vi "load_project.vi"(7 "lv-builder in":refnum<class "lv-builder.lvclass">, 8 "error in (no error)":errorcluster, 11 "project_file":path) -> (0 "error out":errorcluster, 1 "config":T3, 2 "lv-builder out":refnum<class "lv-builder.lvclass">, 3 "build_spec_info []":T1[](array[typedef]), 4 "commit_hash":string)   [LabVIEW 2015, in "lv-build-interface.lvlib"]
uses:
  lv-build-interface.lvlib
  lv-builder/class/lv-builder.lvclass
  lv-build/public/_controls/configuration.ctl
  lv-build/public/_controls/build_specification.ctl
  lv-build/public/_controls/build_type.ctl
  lv-build/public/_controls/configuration_command.ctl
  <userlib>/antonio-alexander/lv-bin/public/api/v1/advanced/add_data_path_single.vi
  lv-build/lv-build.lvlib
  <userlib>/antonio-alexander/lv-bin-git/public/api/v1/v1.lvlib
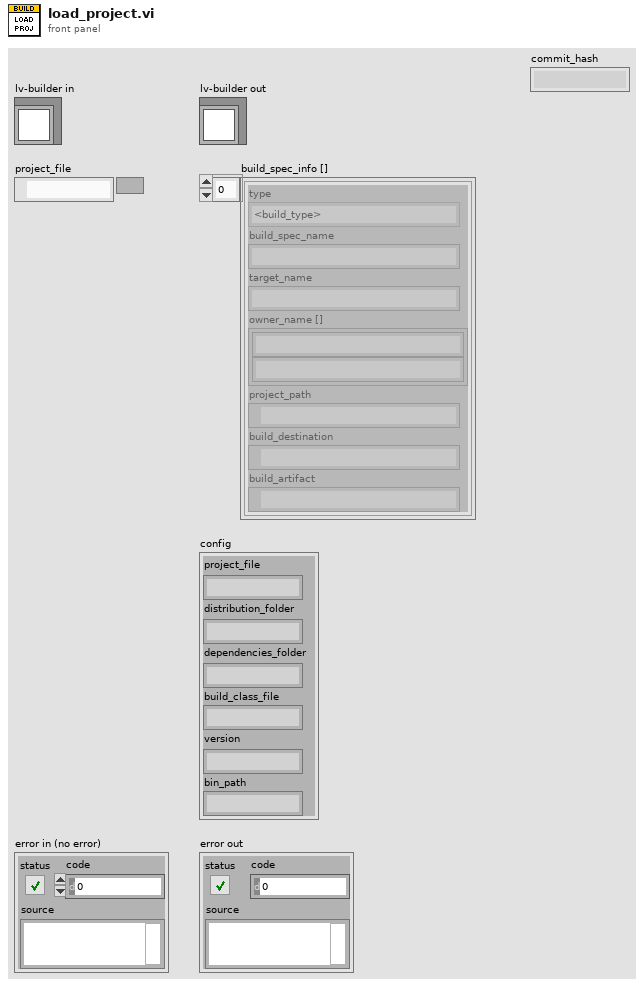
[diagram p1: front panel]
types:
  T1 = typedef "lv-build.lvlib/build_specification.ctl" = cluster{"type":T2, "build_spec_name":string, "target_name":string, "owner_name []":string[], "project_path":path, "build_destination":path, "build_artifact":path}
  T2 = typedef "lv-build.lvlib/build_type.ctl" = enum16{"<build_type>", "application_pc", "application_rt", "installer", "llb", "lvlibp", "zip", "fpga", "<null>"}
  T3 = typedef "lv-build.lvlib/configuration.ctl" = cluster{"project_file":string, "distribution_folder":string, "dependencies_folder":string, "build_class_file":string, "version":string, "bin_path":string}
  T4 = typedef "lv-build.lvlib/configuration_command.ctl" = enum16{"<config_command>", "read_config", "write_config", "<null>"}
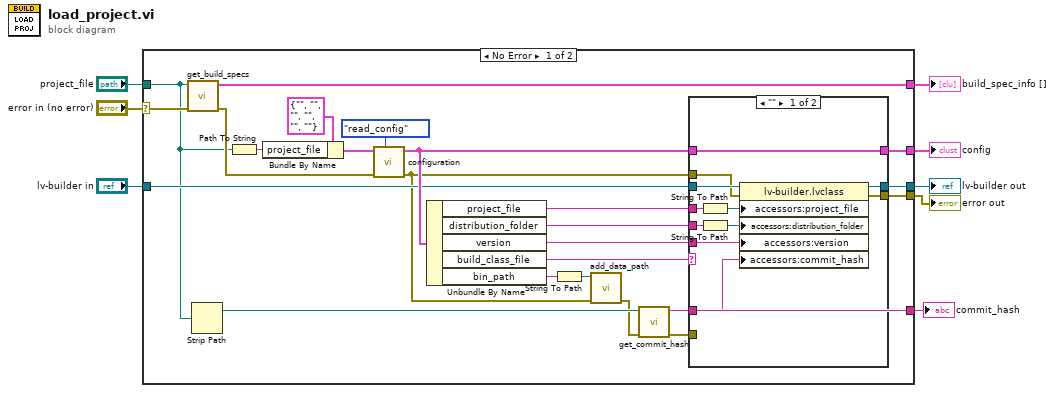
[diagram p0: block diagram]
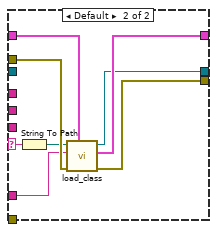
[diagram p2: hidden frame]
diagram:
  n1 = case shown="No Error" "error in (no error)" {
    selector: "error in (no error)" -> [w26 w53]
    tunnel: [w28 _] -> w8
    tunnel: [w24 _] -> w6
    tunnel: [w23 w53] -> w5
    tunnel: [w22 w52] -> w4
    tunnel: "lv-builder in" -> [w20 w52]
    tunnel: "project_file" -> [w19 _]
    tunnel: [w11 _] -> w1
    frame No Error {
      n2 = call "get_build_specs.vi"("error in (no error)"=w26, "project path"=w19) -> ("error out"=w32:errorcluster, "build_spec_info []"=w28:T1[])  [unwired: 8 in]
      n3 = Strip Path(path=w19) -> (stripped path=w18:path)  [unwired: 1 out]
      n4 = Path To String(path=w19) -> (string=w31:string)
      n5 = Bundle By Name(cluster=T3 {"project_file"="", "distribution_folder"="", "dependencies_folder"="", "build_class_file"="", "version"="", "bin_path"=""} ("config in"), "project_file"=w31) -> (w30:T3)
      n6 = call "configuration.vi"("command"=configuration_command."read_config", "error in (no error)"=w32, "config in"=w30) -> ("error out"=w10:errorcluster, "config out"=w25:T3)  [unwired: 7 in]
      n7 = Unbundle By Name(w25) -> ("project_file"=w17:string, "distribution_folder"=w16:string, "version"=w15:string, "build_class_file"=w21:string, "bin_path"=w14:string)
      n8 = String To Path(string=w14) -> (path=w13:path)
      n9 = call-poly <userlib>:"add_data_path.vi"("error in (no error)"=w10, "path_to_add"=w13) -> ("error out"=w12:errorcluster)  [unwired: 9 in]
      n10 = call <userlib>:"get_commit_hash.vi"("error in (no error)"=w12, "path"=w18) -> ("error out"=w9:errorcluster, "commit_hash"=w11:string)  [unwired: 8 in]
      n11 = case shown="\"\"" w21 {
        selector: w21 -> [_ w49]
        tunnel: w25 -> [w43 w50]
        tunnel: w11 -> [w37 w48]
        tunnel: [w43 w47] -> w24
        tunnel: [w34 w46] -> w23
        tunnel: [w41 w45] -> w22
        tunnel: w20 -> [w42 _]
        tunnel: w17 -> [w40 _]
        tunnel: w16 -> [w39 _]
        tunnel: w15 -> [w38 _]
        tunnel: w10 -> [w33 w51]
        tunnel: w9 -> [_ _]
        frame "" {
          n12 = String To Path(string=w40) -> (path=w36:path)
          n13 = String To Path(string=w39) -> (path=w35:path)
          n14 = property class="lv-builder.lvclass"(reference=w42, error in=w33, "accessors:project_file"=w36, "accessors:distribution_folder"=w35, "accessors:version"=w38, "accessors:commit_hash"=w37) -> (reference out=w41:refnum<class "lv-builder.lvclass">, error out=w34:errorcluster)
        }
        frame Default {
          n15 = String To Path(string=w49) -> (path=w44:path)
          n16 = call "load_class.vi"("config in"=w50, "error in (no error)"=w51, "commit_hash"=w48, "lvclass_path"=w44) -> ("error out"=w46:errorcluster, "config out"=w47:T3, "lv-builder"=w45:refnum<class "lv-builder.lvclass">)  [unwired: 5 in]
        }
      }
    }
    frame Error {
    }
  }
  "lv-builder out" <- w4
  "error out" <- w5
  "config" <- w6
  "build_spec_info []" <- w8
  "commit_hash" <- w1
